vi "Error.vi"(10 "Error":errorcluster, 11 "Error in":refnum<class "Error.lvclass">) -> (3 "Error out":refnum<class "Error.lvclass">)   [LabVIEW 2021, in "Error.lvlib" / "Error.lvclass"]
uses:
  Error.lvclass
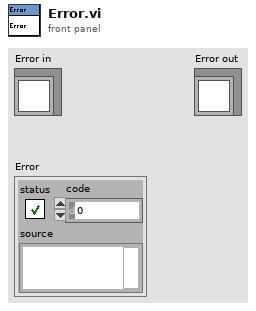
[diagram p1: front panel]
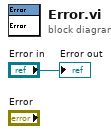
[diagram p0: block diagram]
diagram:
  "Error out" <- "Error in"
